vi "ni579x Validate Mixer Scope.vi"(0 "Register Bus":refnum<class "ni579x Register Bus v1 Host.lvclass">=refnum, 1 "scope":string, 11 "Error In":errorcluster) -> (4 "Register Bus (out)":refnum<class "ni579x Register Bus v1 Host.lvclass">, 15 "Error Out":errorcluster)   [LabVIEW 2015]
uses:
  <instrlib>/ni579x/Register Bus/v1/Host/ni579x Register Bus v1 Host.lvclass
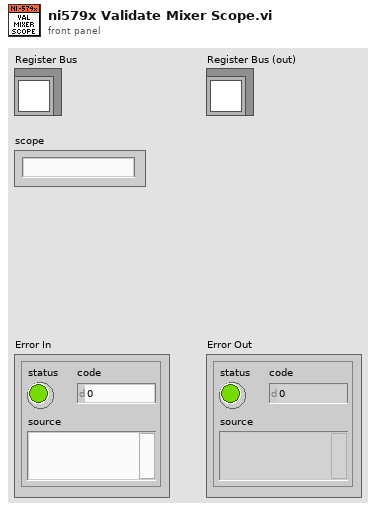
[diagram p1: front panel]
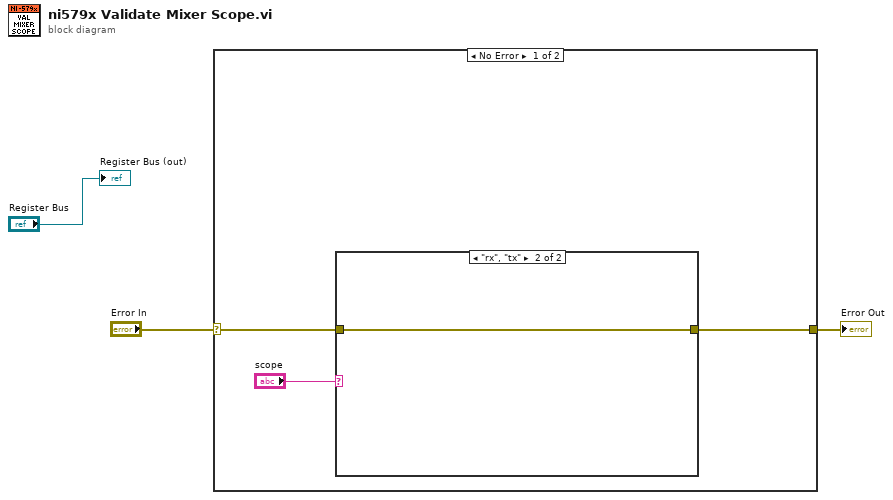
[diagram p0: block diagram]
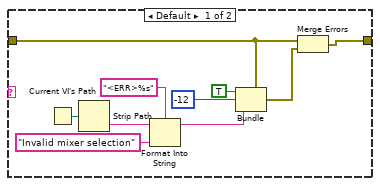
[diagram p2: hidden frame]
diagram:
  n1 = case shown="No Error" "Error In" {
    selector: "Error In" -> [w4 w18]
    tunnel: [w5 w18] -> w2
    frame No Error {
      n2 = case shown="\"rx\", \"tx\"" "scope" {
        tunnel: w4 -> [w9 w17]
        tunnel: [w7 w17] -> w5
        frame Default {
          n3 = Current VI's Path() -> (path=w11:path)
          n4 = Strip Path(path=w11) -> (name=w12:string)  [unwired: 1 out]
          n5 = Format Into String(format string="<ERR>%s", initial string=w12, "Invalid mixer selection" ("input 1")) -> (resulting string=w13:string)  [unwired: 1 in, 1 out]
          n6 = Bundle(cluster=w9, "status"=TRUE, "code"=-12, "source"=w13) -> (w8:errorcluster)
          n7 = Merge Errors(w9, w8) -> (w7:errorcluster)
        }
        frame "rx", "tx" {
        }
      }
    }
    frame Error {
    }
  }
  "Error Out" <- w2
  "Register Bus (out)" <- "Register Bus"
